vi "Read Checked-out.vi"(8 "error in (no error)":errorcluster, 11 "DevInfo in":refnum<class "DevInfo.lvclass">) -> (0 "error out":errorcluster, 2 "Checked-out":bool, 3 "DevInfo out":refnum<class "DevInfo.lvclass">)   [LabVIEW 2016, in "Hardware.lvlib" / "DevInfo.lvclass"]
uses:
  <userlib>/Common Components/Hardware/DevInfo/DevInfo.lvclass
  <userlib>/Common Components/Hardware/DevInfo/DevInfo.lvclass/DevInfo.ctl
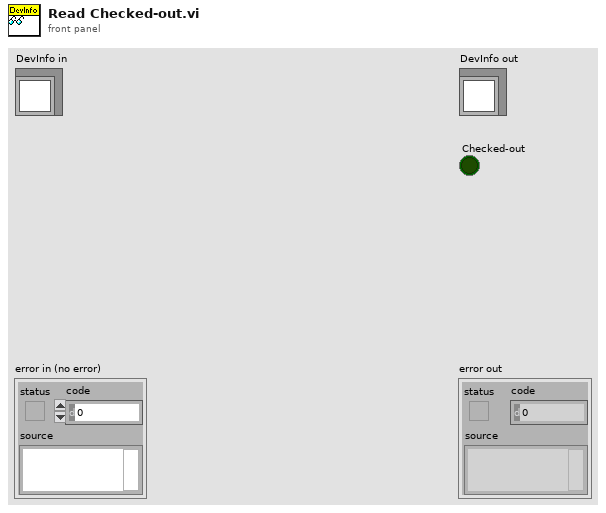
[diagram p1: front panel]
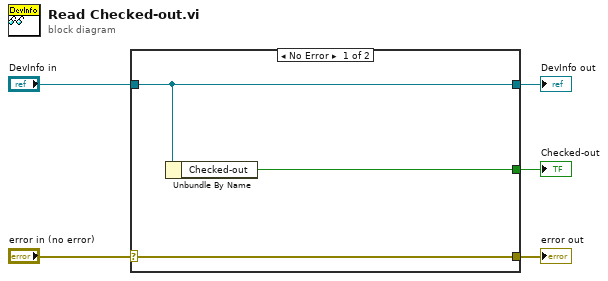
[diagram p0: block diagram]
diagram:
  n1 = case shown="No Error" "error in (no error)" {
    selector: "error in (no error)" -> [w8 w9]
    tunnel: [w8 w9] -> w4
    tunnel: [w7 w10] -> w2
    tunnel: "DevInfo in" -> [w7 w10]
    tunnel: [w6 _] -> w1
    frame No Error {
      n2 = Unbundle By Name(w7) -> ("Checked-out"=w6:bool)
    }
    frame Error {
    }
  }
  "error out" <- w4
  "DevInfo out" <- w2
  "Checked-out" <- w1
